vi "Save file Dialog.vi"(8 "error in (no error)":errorcluster, 10 "Default file name":string caption="default name") -> (0 "error out":errorcluster, 2 "File name":string, 3 "selected path":path)   [LabVIEW 2014]
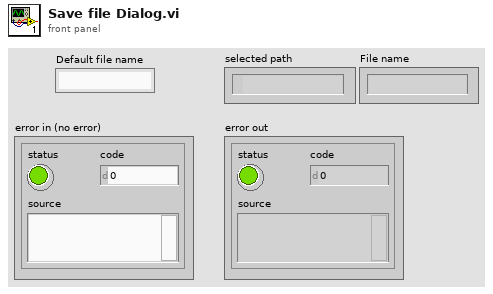
[diagram p1: front panel]
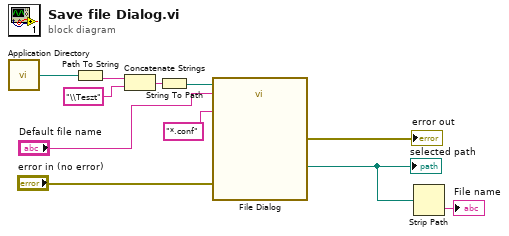
[diagram p0: block diagram]
diagram:
  n1 = call <vilib>:"Application Directory.vi"() -> ("Application Directory"=w2:path)
  n2 = Path To String(path=w2) -> (string=w6:string)
  n3 = Concatenate Strings(w6, "\\Teszt" ("prompt (Choose or enter file path)")) -> (w5:string)
  n4 = String To Path(string=w5) -> (path=w3:path)
  n5 = call "File Dialog"("start path"=w3, "default name"="Default file name", "error in"="error in (no error)", "pattern (all files)"="*.conf") -> ("selected path"=w9:path, "error out"=→"error out":errorcluster)  [unwired: 8 in, 2 out]
  "selected path" <- w9
  n6 = Strip Path(path=w9) -> (name=→"File name":string)  [unwired: 1 out]
